vi "GMLAN Service Broadcast.vi"(6 "error source":string="Diagnostic Service.vi", 8 "error in (no error)":errorcluster, 9 "data in":u8[](array[numeric]), 10 "require response?":bool=TRUE, 11 "diag ref in":T1={"Diag CAN Handle"=0, "Transport Protocol"=enum."ISO TP - Normal Mode", "Receive Address Extension"=0, "Transmit Address Extension"=0, "Receive CAN Id"=0, "Transmit CAN Id"=0, "Log Frames ?"=FALSE, "My TP Address"=0, "Other TP Address"=0, "T1"=0, "T2"=0, "T3"=0, "T4"=0, "Tx SN"=0, "Block Size"=0, "Rx SN"=0, "VW TP Initialized?"=FALSE, "Tx block no"=0, "baud rate"=0, "Interface"="", "Channel Diag CAN Handle"=0, "UDP Connection ID"=refnum, "TCP Connection ID"=refnum, "Target IP Addr"=0, "Source Address"=0, "Target Address"=0, "Send Header NACK?"=FALSE, "DLL Handle"=0, "NAD"=0, "Time Stamp read first"=0.0, "Time Stamp read last"=0.0, "Time Stamp write first"=0.0, "Time Stamp write last"=0.0, "Time Stamp write"=0.0, "Time Stamp read"=0.0, " I/O Mode"=0, "FD Baudrate"=0, "TX_DL"=8, "RX_DL"=8, "DoIP Protocol Version"=1, " Selected I/O Mode"=0, "TesterPresent Counter"=0, "TesterPresent Limit"=0, "TesterPresent Tick[ms]"=10, "TesterPresent RequireResponse?"=FALSE, "TesterPresent Stored Ref?"=FALSE, "TesterPresent Message"=[], "TesterPresent Task Handle"=0, "TesterPresent Semaphore"=refnum, "Response Plausibility Check"=1, "Default Version?"=TRUE, "Diagostic Globals"={"Timeout FC (Bs)"=250, "Timeout CF (Cr)"=250, "Timeout Diag Command"=1000, "Receive Block Size (BS)"=0, "Wait Time CF (STmin)"=5, "Max Waits (N_WFTmax)"=10, "Waits to Send (N_WAIT)"=0, "Time between Waits (TW)"=25, "Fill CAN Frames?"=TRUE, "Fill Byte"=255, "Invalid Response as Error?"=FALSE, "Max RspPending Count"=5, "VWTP Command Timeout"=50, "Transport Protocol"=enum."Diagnostics on IP", "Diag CAN Handle"=0, "DLL Handle"=0, "Timeout RspPending"=1000}, "Session-based Properties?"=FALSE} {"Diagostic Globals"."Fill Byte" format="%x"; "TesterPresent Message" format="%.0x"; "Selected I/O Mode" items=["CAN", "CAN FD", "CAN FD+BRS", "ECU Determined"]; "DoIP Protocol Version" items=["2010"=1, "2012"=2]; "RX_DL" items=["8"=8, "12"=12, "16"=16, "20"=20, "24"=24, "32"=32, "48"=48, "64"=64]; "TX_DL" items=["8"=8, "12"=12, "16"=16, "20"=20, "24"=24, "32"=32, "48"=48, "64"=64]; "I/O Mode" items=["CAN", "CAN FD", "CAN FD+BRS", "Not yet determined"]}) -> (0 "error out":errorcluster, 1 "data out":u8[](array[numeric]), 2 "error code":u8, 3 "diag ref out":T1={"Diag CAN Handle"=0, "Transport Protocol"=enum."ISO TP - Normal Mode", "Receive Address Extension"=0, "Transmit Address Extension"=0, "Receive CAN Id"=0, "Transmit CAN Id"=0, "Log Frames ?"=FALSE, "My TP Address"=0, "Other TP Address"=0, "T1"=0, "T2"=0, "T3"=0, "T4"=0, "Tx SN"=0, "Block Size"=0, "Rx SN"=0, "VW TP Initialized?"=FALSE, "Tx block no"=0, "baud rate"=0, "Interface"="", "Channel Diag CAN Handle"=0, "UDP Connection ID"=refnum, "TCP Connection ID"=refnum, "Target IP Addr"=0, "Source Address"=0, "Target Address"=0, "Send Header NACK?"=FALSE, "DLL Handle"=0, "NAD"=0, "Time Stamp read first"=0.0, "Time Stamp read last"=0.0, "Time Stamp write first"=0.0, "Time Stamp write last"=0.0, "Time Stamp write"=0.0, "Time Stamp read"=0.0, " I/O Mode"=0, "FD Baudrate"=0, "TX_DL"=8, "RX_DL"=8, "DoIP Protocol Version"=1, " Selected I/O Mode"=0, "TesterPresent Counter"=0, "TesterPresent Limit"=0, "TesterPresent Tick[ms]"=10, "TesterPresent RequireResponse?"=FALSE, "TesterPresent Stored Ref?"=FALSE, "TesterPresent Message"=[], "TesterPresent Task Handle"=0, "TesterPresent Semaphore"=refnum, "Response Plausibility Check"=1, "Default Version?"=TRUE, "Diagostic Globals"={"Timeout FC (Bs)"=250, "Timeout CF (Cr)"=250, "Timeout Diag Command"=1000, "Receive Block Size (BS)"=0, "Wait Time CF (STmin)"=5, "Max Waits (N_WFTmax)"=10, "Waits to Send (N_WAIT)"=0, "Time between Waits (TW)"=25, "Fill CAN Frames?"=TRUE, "Fill Byte"=255, "Invalid Response as Error?"=FALSE, "Max RspPending Count"=5, "VWTP Command Timeout"=50, "Transport Protocol"=enum."Diagnostics on IP", "Diag CAN Handle"=0, "DLL Handle"=0, "Timeout RspPending"=1000}, "Session-based Properties?"=FALSE} {"Diagostic Globals"."Fill Byte" format="%x"; "TesterPresent Message" format="%.0x"; "Selected I/O Mode" items=["CAN", "CAN FD", "CAN FD+BRS", "ECU Determined"]; "DoIP Protocol Version" items=["2010"=1, "2012"=2]; "RX_DL" items=["8"=8, "12"=12, "16"=16, "20"=20, "24"=24, "32"=32, "48"=48, "64"=64]; "TX_DL" items=["8"=8, "12"=12, "16"=16, "20"=20, "24"=24, "32"=32, "48"=48, "64"=64]; "I/O Mode" items=["CAN", "CAN FD", "CAN FD+BRS", "Not yet determined"]})   [LabVIEW 2019, in "GMLAN.lvlib"]
uses:
  GMLAN.lvlib
  <vilib>/Automotive Diagnostic Command Set/Diagnostic Transport.llb/Diag Reference.ctl
  <vilib>/Automotive Diagnostic Command Set/Diagnostic Transport.llb/Transport Protocol Selector.ctl
  <vilib>/Automotive Diagnostic Command Set/Diagnostic Transport.llb/DoIP Protocol Version.ctl
  <vilib>/Automotive Diagnostic Command Set/Diagnostic Transport.llb/Diag Globals.ctl
  <vilib>/Automotive Diagnostic Command Set/Diagnostic Transport.llb/ISOTP Transmit.vi
  <vilib>/Automotive Diagnostic Command Set/Diagnostic Transport.llb/ISOTP7 Transmit.vi
  <vilib>/Automotive Diagnostic Command Set/Diagnostic Transport.llb/DoIP Transmit.vi
  <vilib>/Automotive Diagnostic Command Set/Diagnostic Transport.llb/LIN ISOTP Transmit.vi
  <vilib>/Automotive Diagnostic Command Set/Diagnostic Transport.llb/Diagnostic Service Recv.vi
  <vilib>/Automotive Diagnostic Command Set/Diagnostic Transport.llb/ISOTP Send FF.vi
  <vilib>/Automotive Diagnostic Command Set/Diagnostic Transport.llb/ISOTP Send CFs.vi
  <vilib>/Automotive Diagnostic Command Set/Diagnostic Transport.llb/ISOTP Send Frame.vi
  <vilib>/Automotive Diagnostic Command Set/Diagnostic Transport.llb/ISOTP7 Send FF.vi
  <vilib>/Automotive Diagnostic Command Set/Diagnostic Transport.llb/ISOTP7 Send CFs.vi
  <vilib>/Automotive Diagnostic Command Set/Diagnostic Transport.llb/ISOTP7 Send Frame.vi
  <vilib>/Automotive Diagnostic Command Set/Diagnostic Transport.llb/DoIP TCP Msg Send.vi
  <vilib>/Automotive Diagnostic Command Set/Diagnostic Transport.llb/DoIP TCP Msg Recv.vi
  <vilib>/Automotive Diagnostic Command Set/Diagnostic Transport.llb/DoIP Check Addresses.vi
  <vilib>/Automotive Diagnostic Command Set/Diagnostic Transport.llb/DoIP Check ACK Code.vi
  <vilib>/Automotive Diagnostic Command Set/Diagnostic Transport.llb/ISOTP Receive.vi
  <vilib>/Automotive Diagnostic Command Set/Diagnostic Transport.llb/ISOTP7 Receive.vi
  <vilib>/Automotive Diagnostic Command Set/Diagnostic Transport.llb/DoIP Receive.vi
  <vilib>/Automotive Diagnostic Command Set/Diagnostic Transport.llb/LIN ISOTP Receive.vi
  <vilib>/Automotive Diagnostic Command Set/Diagnostic Transport.llb/Diag Get Globals.vi
  <vilib>/Automotive Diagnostic Command Set/Diagnostic Transport.llb/ISOTP Recv FC.vi
  <vilib>/Automotive Diagnostic Command Set/Diagnostic Transport.llb/ISOTP Send CF.vi
  <vilib>/Automotive Diagnostic Command Set/Diagnostic Transport.llb/Diag Fill Frame.vi
  <vilib>/Automotive Diagnostic Command Set/Diagnostic Transport.llb/ISOTP Calc Send Params.vi
  <vilib>/Automotive Diagnostic Command Set/Diagnostic Transport.llb/ISOTP7 Recv FC.vi
  <vilib>/Automotive Diagnostic Command Set/Diagnostic Transport.llb/ISOTP7 Send CF.vi
  <vilib>/Automotive Diagnostic Command Set/Diagnostic Transport.llb/DoIP Add Addresses.vi
  <vilib>/Automotive Diagnostic Command Set/Diagnostic Transport.llb/DoIP TCP Send.vi
  <vilib>/Automotive Diagnostic Command Set/Diagnostic Transport.llb/DoIP TCP Recv.vi
  <vilib>/Automotive Diagnostic Command Set/Diagnostic Transport.llb/DoIP Add Header.vi
  <vilib>/Automotive Diagnostic Command Set/Diagnostic Transport.llb/ISOTP Recv Frame.vi
  <vilib>/Automotive Diagnostic Command Set/Diagnostic Transport.llb/ISOTP Recv CFs.vi
  <vilib>/Automotive Diagnostic Command Set/Diagnostic Transport.llb/ISOTP7 Recv Frame.vi
  <vilib>/Automotive Diagnostic Command Set/Diagnostic Transport.llb/ISOTP7 Recv CFs.vi
  <vilib>/Automotive Diagnostic Command Set/Diagnostic Transport.llb/DoIP Send Alive.vi
  <vilib>/Automotive Diagnostic Command Set/Diagnostic Transport.llb/DoIP Check Error.vi
  <vilib>/Automotive Diagnostic Command Set/Diagnostic Transport.llb/ISOTP Check Redo.vi
  <vilib>/Automotive Diagnostic Command Set/Diagnostic Transport.llb/ISOTP Recv Block.vi
  <vilib>/Automotive Diagnostic Command Set/Diagnostic Transport.llb/ISOTP7 Recv Block.vi
  <vilib>/Utility/error.llb/Clear Errors.vi
  <vilib>/Automotive Diagnostic Command Set/Diagnostic Transport.llb/ISOTP Send FC.vi
  <vilib>/Automotive Diagnostic Command Set/Diagnostic Transport.llb/ISOTP Add CF.vi
  <vilib>/Automotive Diagnostic Command Set/Diagnostic Transport.llb/ISOTP7 Send FC.vi
  <vilib>/Automotive Diagnostic Command Set/Diagnostic Transport.llb/ISOTP7 Add CF.vi
  <vilib>/Automotive Diagnostic Command Set/Diagnostic Transport.llb/Diag Globals.vi
  <vilib>/Automotive Diagnostic Command Set/Diagnostic Transport.llb/CAN Send Frame Check Queue.vi
  <vilib>/Automotive Diagnostic Command Set/Diagnostic Transport.llb/Diag CAN get timestamp.vi
  <vilib>/Automotive Diagnostic Command Set/Diagnostic Transport.llb/Diag CAN read.vi
  <vilib>/Automotive Diagnostic Command Set/Diagnostic Transport.llb/ISOTP Calc Actual IO Mode.vi
  <vilib>/Automotive Diagnostic Command Set/Diagnostic Transport.llb/ISOTP Get FC Data.vi
  <vilib>/Automotive Diagnostic Command Set/Diagnostic Transport.llb/VWTP Write.vi
  <vilib>/Automotive Diagnostic Command Set/Diagnostic Transport.llb/DoIP Analyze Header.vi
  <vilib>/Automotive Diagnostic Command Set/Diagnostic Transport.llb/Diag CAN status.vi
  <vilib>/Automotive Diagnostic Command Set/Diagnostic Transport.llb/VWTP Read.vi
  <vilib>/addons/Automotive Diagnostic Command Set/NI_Automotive Diagnostic Command Set.lvlib
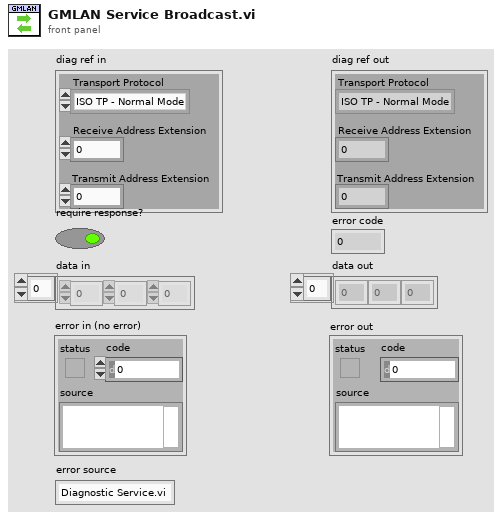
[diagram p1: front panel]
types:
  T1 = typedef "NI_Automotive Diagnostic Command Set.lvlib/Diag Reference.ctl" = cluster{"Diag CAN Handle":u32, "Transport Protocol":T2, "Receive Address Extension":u8, "Transmit Address Extension":u8, "Receive CAN Id":u32, "Transmit CAN Id":u32, "Log Frames ?":bool, "My TP Address":u8, "Other TP Address":u8, "T1":u16, "T2":u16, "T3":u16, "T4":u16, "Tx SN":u8, "Block Size":u8, "Rx SN":u8, "VW TP Initialized?":bool, "Tx block no":u8, "baud rate":u64, "Interface":string, "Channel Diag CAN Handle":u32, "UDP Connection ID":refnum<k16>, "TCP Connection ID":refnum<k5>, "Target IP Addr":u32, "Source Address":u16, "Target Address":u16, "Send Header NACK?":bool, "DLL Handle":u32, "NAD":u8, "Time Stamp read first":dbl, "Time Stamp read last":dbl, "Time Stamp write first":dbl, "Time Stamp write last":dbl, "Time Stamp write":dbl, "Time Stamp read":dbl, " I/O Mode":u32, "FD Baudrate":u64, "TX_DL":u16, "RX_DL":u16, "DoIP Protocol Version":T3, " Selected I/O Mode":u32, "TesterPresent Counter":u32, "TesterPresent Limit":u32, "TesterPresent Tick[ms]":i32, "TesterPresent RequireResponse?":bool, "TesterPresent Stored Ref?":bool, "TesterPresent Message":u8[], "TesterPresent Task Handle":i32, "TesterPresent Semaphore":T4, "Response Plausibility Check":u32, "Default Version?":bool, "Diagostic Globals":T5, "Session-based Properties?":bool}
  T2 = typedef "NI_Automotive Diagnostic Command Set.lvlib/Transport Protocol Selector.ctl" = enum16{"ISO TP - Normal Mode", "ISO TP - Mixed Mode", "VW TP 2.0", "Diagnostics on IP", "ISO TP LIN"}
  T3 = typedef "NI_Automotive Diagnostic Command Set.lvlib/DoIP Protocol Version.ctl" = u8
  T4 = typedef "Semaphore RefNum" = refnum<k1>
  T5 = typedef "NI_Automotive Diagnostic Command Set.lvlib/Diag Globals.ctl" = cluster{"Timeout FC (Bs)":u32, "Timeout CF (Cr)":u32, "Timeout Diag Command":u32, "Receive Block Size (BS)":u8, "Wait Time CF (STmin)":u8, "Max Waits (N_WFTmax)":u8, "Waits to Send (N_WAIT)":i32, "Time between Waits (TW)":u32, "Fill CAN Frames?":bool, "Fill Byte":u32, "Invalid Response as Error?":bool, "Max RspPending Count":u32, "VWTP Command Timeout":u32, "Transport Protocol":T2, "Diag CAN Handle":u32, "DLL Handle":u32, "Timeout RspPending":u32}
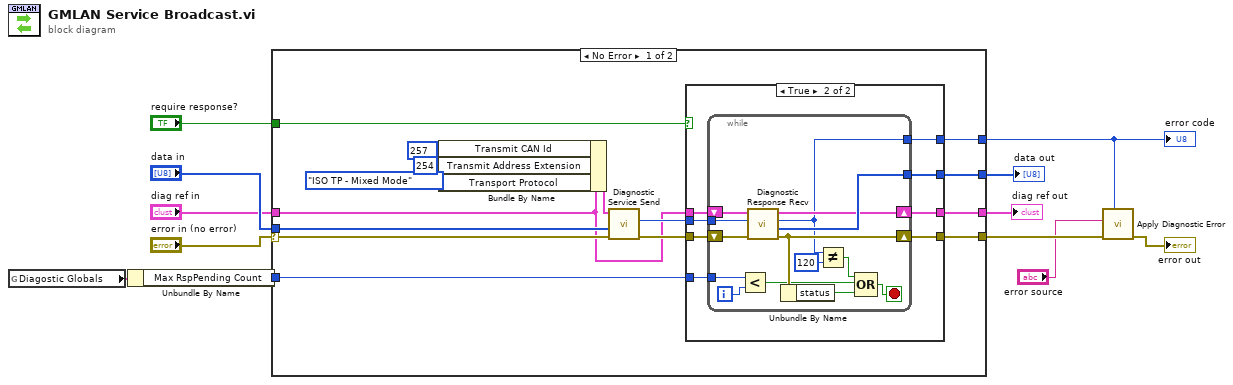
[diagram p0: block diagram]
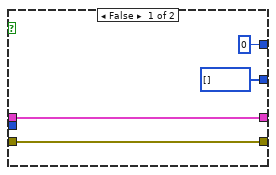
[diagram p2: hidden frame]
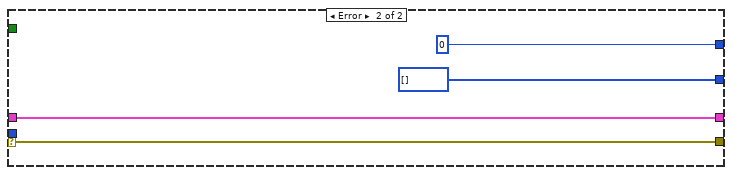
[diagram p3: hidden frame]
diagram:
  n1 = global read "Diag Globals.vi" "Diagostic Globals"() -> (w4:T5)
  n2 = Unbundle By Name(w4) -> ("Max RspPending Count"=w3:u32)
  n3 = case shown="No Error" "error in (no error)" {
    selector: "error in (no error)" -> [w21 w56]
    tunnel: "data in" -> [w27 _]
    tunnel: [w26 u8[] [] ("data out")] -> w11
    tunnel: [w13 w57] -> w1
    tunnel: [w25 w56] -> w10
    tunnel: "diag ref in" -> [w14 w57]
    tunnel: [w22 u8 0 ("error code")] -> w7
    tunnel: "require response?" -> [w20 _]
    tunnel: w3 -> [w19 _]
    frame No Error {
      n4 = Bundle By Name(cluster=w14, "Transmit CAN Id"=u32 257 ("Transmit Address Extension"), "Transmit Address Extension"=u8 254, "Transport Protocol"=Transport_Protocol_Selector."ISO TP - Mixed Mode") -> (w15:T1)
      n5 = call <vilib>:"Diagnostic Service Send.vi"("error in (no error)"=w21, "data in"=w27, "diag ref in"=w15) -> ("error out"=w24:errorcluster, "service id"=w23:u8)  [unwired: 7 out]
      n6 = case shown="True" w20 {
        tunnel: [u8[] [] ("data out") w39] -> w26
        tunnel: [w30 w33] -> w13
        tunnel: [w29 w38] -> w25
        tunnel: w14 -> [w30 w32]
        tunnel: w24 -> [w29 w37]
        tunnel: w23 -> [_ w36]
        tunnel: [u8 0 ("error code") w35] -> w22
        tunnel: w19 -> [_ w34]
        frame False {
        }
        frame True {
          n7 = while {
            tunnel: [w53] -> w39
            tunnel: w36 -> [w50]
            shift-right: [w49] -> w38
            shift-left: w37 -> [w51]
            tunnel: [w44] -> w35
            shift-right: [w45] -> w33
            shift-left: w32 -> [w52]
            tunnel: w34 -> [w40]
            i -> [w42]
            stop <- w47 stop-if-true
            n8 = Less?(x=w40, y=w42) -> (x < y?=w41:bool)
            n9 = call <vilib>:"Diagnostic Response Recv.vi"("error in (no error)"=w51, "service id"=w50, "diag ref in"=w52) -> ("error out"=w49:errorcluster, "data out"=w53:u8[], "error code"=w44:u8, "diag ref out"=w45:T1)  [unwired: 1 in, 4 out]
            n10 = Unbundle By Name(w49) -> ("status"=w46:bool)
            n11 = Not Equal?(x=w44, y=u8 120) -> (x != y?=w43:bool)
            n12 = Compound Arithmetic op=OR(w43, w41, w46) -> (w47:bool)
          }
        }
      }
    }
    frame Error {
    }
  }
  "data out" <- w11
  "error code" <- w7
  "diag ref out" <- w1
  n13 = call <vilib>:"Apply Diagnostic Error.vi"("error code"=w7, "error in (no error)"=w10, "error source"="error source") -> ("error out"=→"error out":errorcluster)  [unwired: 8 out]
